vi "Initialize app.vi"(8 "error in (no error)":errorcluster) -> (0 "error out":errorcluster)   [LabVIEW 2019, in "Shared.lvlib"]
uses:
  Shared.lvlib
  App INI data.ctl
  <vilib>/Utility/sysdir.llb/System Directory Type.ctl
  System GV.vi
  <vilib>/Utility/config.llb/NI_LVConfig.lvlib
panel:
  out "system directory":path
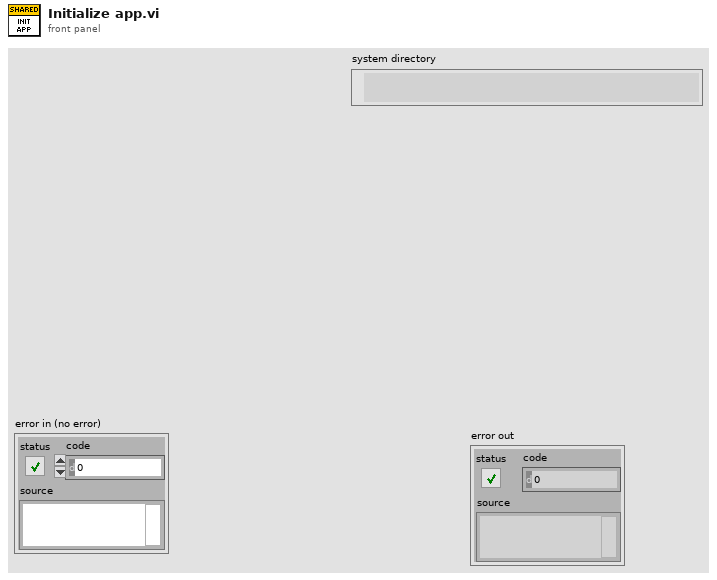
[diagram p1: front panel]
types:
  T1 = typedef "System Directory Type.ctl" = i32
  T2 = typedef "Shared.lvlib/App INI data.ctl" = cluster{"HW INI path":path, "System ID":string, "Log root":path, "PID path":path, "ZMQ port":string}
  T3 = typedef "NI_LVConfig.lvlib/Config Data RefNum.ctl" = refnum<k1>
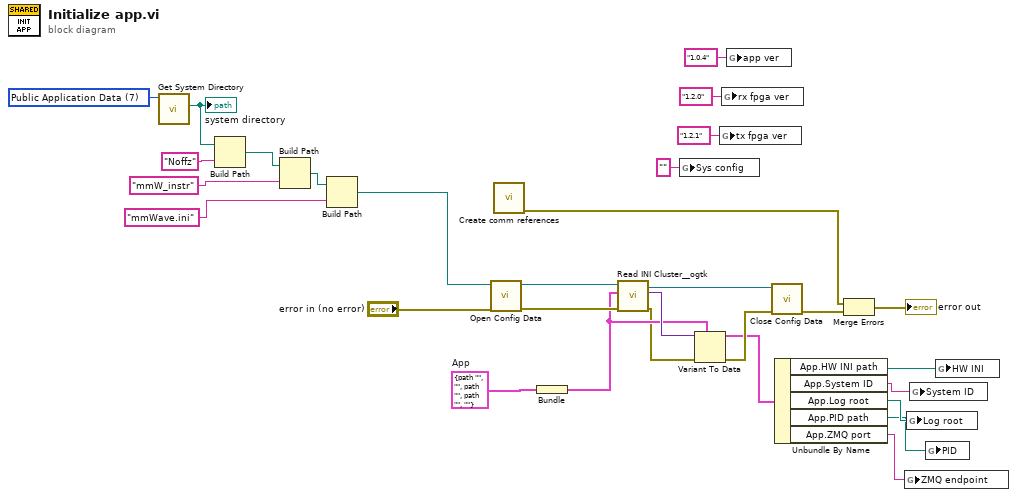
[diagram p0: block diagram]
diagram:
  w16 = T1 7 items=["User Home"=0, "User Desktop"=1, "User Documents"=2, "User Application Data"=3, "User Preferences"=4, "User Temporary"=5, "Public Documents"=6, "Public Application Data"=7, "Public Preferences"=8, "Public Cache"=13, "System Core Libraries"=9, "System Installed Libraries"=10, "Application Files"=11, "Boot Volume Root"=12] ("system directory type")
  w8 = T2 {"HW INI path"=path "", "System ID"="", "Log root"=path "", "PID path"=path "", "ZMQ port"=""}  # App
  n1 = call <vilib>:"Get System Directory.vi"("system directory type"=w16) -> ("system directory"=w15:path)  [unwired: 10 in]
  "system directory" <- w15
  n2 = Build Path(base path=w15, name or relative path="Noffz") -> (appended path=w14:path)
  n3 = Build Path(base path=w14, name or relative path="mmW_instr") -> (appended path=w11:path)
  n4 = Build Path(base path=w11, name or relative path="mmWave.ini") -> (appended path=w9:path)
  n5 = call <vilib>:"Open Config Data.vi"("error in (no error)"="error in (no error)", "configuration file path"=w9) -> ("error out"=w29:errorcluster, "refnum"=w30:T3)  [unwired: 7 in, 1 out]
  n6 = call "Create comm references.vi"() -> ("error out"=w17:errorcluster)  [unwired: 11 in]
  n7 = Bundle("App"=w8) -> (w24:cluster{"App":T2})  [unwired: 1 in]
  n8 = call <userlib>:"Read INI Cluster__ogtk.vi"("error in (no error)"=w29, "INI Fomatted Cluster Type"=w24, "refnum"=w30) -> ("error out"=w23:errorcluster, "INI Fomatted Cluster"=w25:variant, "dup refnum"=w27:T3)  [unwired: 4 in, 2 out]
  n9 = global write "System GV.vi" "Sys config"("" ("Sys config")) -> ()
  n10 = Variant To Data(error in=w23, type=w24, Variant=w25) -> (data=w21:cluster{"App":T2}, error out=w22:errorcluster)
  n11 = global write "System GV.vi" "tx fpga ver"("1.2.1" ("tx fpga ver")) -> ()
  n12 = global write "System GV.vi" "rx fpga ver"("1.2.0" ("rx fpga ver")) -> ()
  n13 = global write "System GV.vi" "app ver"("1.0.4" ("app ver")) -> ()
  n14 = call <vilib>:"Close Config Data.vi"("error in (no error)"=w22, "refnum"=w27) -> ("error out"=w26:errorcluster)  [unwired: 8 in, 1 out]
  n15 = Unbundle By Name(w21) -> ("App.HW INI path"=w20:path, "App.System ID"=w19:string, "App.Log root"=w7:path, "App.PID path"=w6:path, "App.ZMQ port"=w1:string)
  n16 = Merge Errors(w17, w26) -> (→"error out":errorcluster)
  n17 = global write "System GV.vi" "ZMQ endpoint"(w1) -> ()
  n18 = global write "System GV.vi" "Log root"(w7) -> ()
  n19 = global write "System GV.vi" "System ID"(w19) -> ()
  n20 = global write "System GV.vi" "PID"(w6) -> ()
  n21 = global write "System GV.vi" "HW INI"(w20) -> ()
